vi "CheckAlarms.vi"(8 "error in (no error)":errorcluster, 11 "Cluster":T1={"Requests"=[], "Limits"={"AckLimit"=2.0, "CompleteLimit"=5.0}}) -> (0 "error out":errorcluster, 2 "JSON string":string, 3 "Requests Out":T1={"Requests"=[], "Limits"={"AckLimit"=2.0, "CompleteLimit"=5.0}})   [LabVIEW 2015]
uses:
  TypeDef/RequestStateCluster.ctl
  LVClasses/Request/Request.lvclass
  LVClasses/Request/Request.lvclass/Request.ctl
  LVClasses/Request/Write Active Alarm.vi
  LVClasses/Request/Read Alarm.vi
  LVClasses/Request/Read RequestID.vi
  LVClasses/Request/Write Alarm.vi
  LVClasses/Request/Read StartTime.vi
  LVClasses/Request/Read AckTime.vi
  LVClasses/Request/Read FulfilledTime.vi
  Database/DatabaseApi.lvlib
panel:
  out "Time Dif":dbl
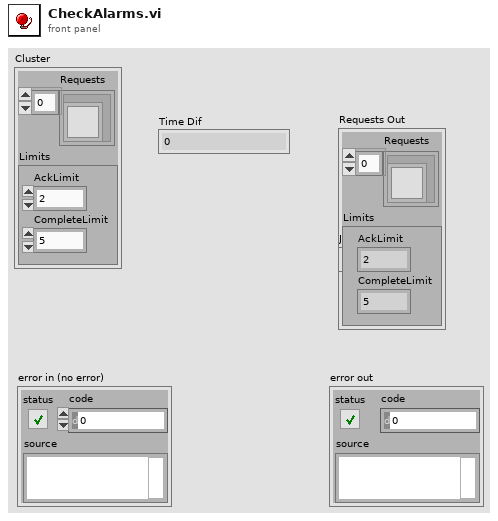
[diagram p1: front panel]
types:
  T1 = typedef "RequestStateCluster.ctl" = cluster{"Requests":refnum<class "Request.lvclass">[], "Limits":cluster{"AckLimit":dbl, "CompleteLimit":dbl}}
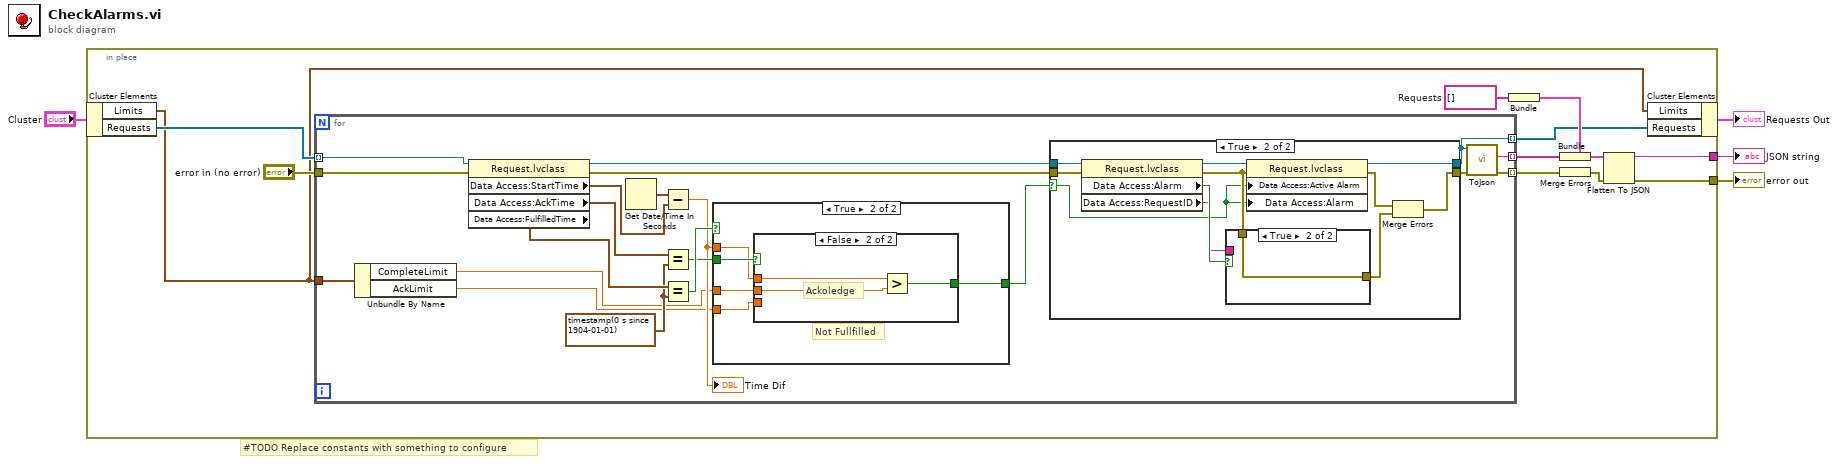
[diagram p0: block diagram]
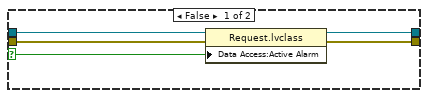
[diagram p2: hidden frame]
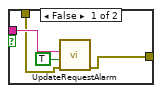
[diagram p3: hidden frame]
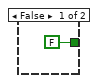
[diagram p4: hidden frame]
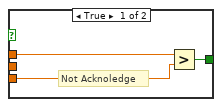
[diagram p5: hidden frame]
diagram:
  # "#TODO Replace constants with something to configure"
  n1 = in-place {
    in-place-border: [w13] -> w4
    in-place-border: [w11] -> w3
    w9 = string[] []  # Requests
    n2 = in-place-cluster #1("Cluster") -> ("Limits"=w5:cluster{"AckLimit":dbl, "CompleteLimit":dbl}, "Requests"=w7:refnum<class "Request.lvclass">[])
    n3 = for {
      tunnel: w7 -> [w36] mode=indexing
      tunnel: [w35] -> w15 mode=indexing
      tunnel: "error in (no error)" -> [w32]
      tunnel: [w34] -> w16 mode=indexing
      tunnel: [w21] -> w6 mode=indexing
      tunnel: w5 -> [w20]
      w27 = timestamp(0 s since 1904-01-01) ("y")
      n4 = Unbundle By Name(w20) -> ("CompleteLimit"=w18:dbl, "AckLimit"=w19:dbl)
      n5 = property class="Request.lvclass"(reference=w36, error in=w32) -> (reference out=w33:refnum<class "Request.lvclass">, error out=w31:errorcluster, "Data Access:StartTime"=w23:timestamp, "Data Access:AckTime"=w29:timestamp, "Data Access:FulfilledTime"=w28:timestamp)
      n6 = Get Date/Time In Seconds() -> (seconds since 1Jan1904=w24:timestamp)
      n7 = Subtract(x=w24, y=w23) -> (x-y=w22:dbl)
      "Time Dif" <- w22
      n8 = Equal?(x=w29, y=w27) -> (x = y?=w25:bool)
      n9 = Equal?(x=w28, y=w27) -> (x = y?=w26:bool)
      n10 = case shown="True" w26 {
        tunnel: w25 -> [_ w63]
        tunnel: w22 -> [_ w62]
        tunnel: [FALSE w61] -> w17
        tunnel: w19 -> [_ w60]
        tunnel: w18 -> [_ w59]
        frame False {
        }
        frame True {
          # "Not Fullfilled"
          n11 = case shown="False" w63 {
            tunnel: w62 -> [w66 w69]
            tunnel: [w65 w68] -> w61
            tunnel: w60 -> [w64 _]
            tunnel: w59 -> [_ w67]
            frame True {
              # "Not Acknoledge"
              n12 = Greater?(x=w66, y=w64) -> (0:w65:bool)
            }
            frame False {
              # "Ackoledge"
              n13 = Greater?(x=w69, y=w67) -> (0:w68:bool)
            }
          }
        }
      }
      n14 = case shown="True" w17 {
        selector: w17 -> [w37 w42]
        tunnel: w33 -> [w41 w52]
        tunnel: w31 -> [w40 w49]
        tunnel: [w39 w44] -> w30
        tunnel: [w38 w51] -> w21
        frame False {
          n15 = property class="Request.lvclass"(reference=w41, error in=w40, "Data Access:Active Alarm"=w37) -> (reference out=w38:refnum<class "Request.lvclass">, error out=w39:errorcluster)
        }
        frame True {
          n16 = property class="Request.lvclass"(reference=w52, error in=w49) -> (reference out=w50:refnum<class "Request.lvclass">, error out=w46:errorcluster, "Data Access:Alarm"=w48:bool, "Data Access:RequestID"=w47:string)
          n17 = case shown="True" w48 {
            tunnel: w47 -> [w56 _]
            tunnel: w46 -> [w54 w57]
            tunnel: [w53 w57] -> w43
            frame False {
              n18 = call "UpdateRequestAlarm.vi"("error in"=w54, "Alarm"=TRUE, "RequestID"=w56) -> ("error out"=w53:errorcluster)  [unwired: 8 in]
            }
            frame True {
            }
          }
          n19 = property class="Request.lvclass"(reference=w50, error in=w46, "Data Access:Active Alarm"=w42, "Data Access:Alarm"=w42) -> (reference out=w51:refnum<class "Request.lvclass">, error out=w45:errorcluster)
          n20 = Merge Errors(w45, w43) -> (w44:errorcluster)
        }
      }
      n21 = call "ToJson.vi"("error in (no error)"=w30, "Request"=w21) -> ("error out"=w34:errorcluster, "Request"=w35:string)  [unwired: 8 in]
    }
    n22 = Bundle("Requests"=w9) -> (w8:cluster{"Requests":string[]})  [unwired: 1 in]
    n23 = Bundle(cluster=w8, "Requests"=w15) -> (w10:cluster{"Requests":string[]})
    n24 = Merge Errors(w16) -> (w14:errorcluster)
    n25 = Flatten To JSON(anything=w10, error in (no error)=w14) -> (JSON string=w11:string, 11:w13:errorcluster)  [unwired: 1 in]
    n26 = in-place-cluster #1("Limits"=w5, "Requests"=w6) -> (→"Requests Out":T1)
  }
  "error out" <- w4
  "JSON string" <- w3
